vi "GEOM_VAR_RequestedROIsArray.vi"(9 "Action":T2, 10 "ROIs":T1[](array[typedef])) -> (2 "ROIs out":T1[](array[typedef]))   [LabVIEW 2016]
uses:
  GEOM_VAR_action.ctl
  GEOM_Coords.ctl
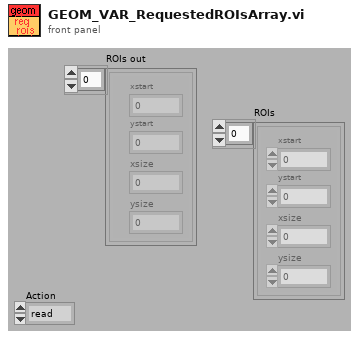
[diagram p1: front panel]
types:
  T1 = typedef "GEOM_Coords.ctl" = cluster{"xstart":u32, "ystart":u32, "xsize":u32, "ysize":u32}
  T2 = typedef "GEOM_VAR_action.ctl" = enum16{"read", "write"}
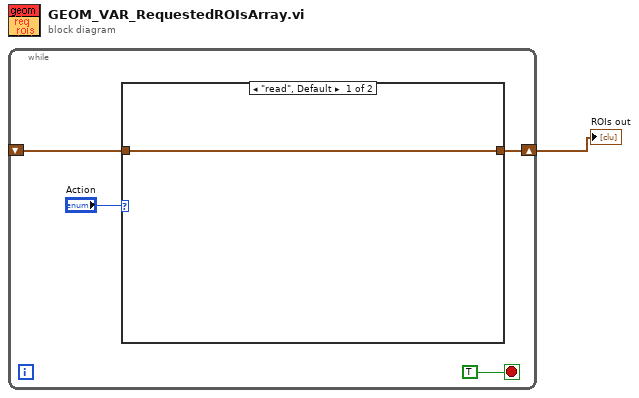
[diagram p0: block diagram]
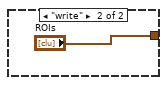
[diagram p2: hidden frame]
diagram:
  n1 = while {
    shift-right: [w2] -> w1
    shift-left: _ -> [w4]
    stop <- TRUE stop-if-true
    n2 = case shown="\"read\", Default" "Action" {
      tunnel: w4 -> [w6 _]
      tunnel: [w6 "ROIs"] -> w2
      frame "read", Default {
      }
      frame "write" {
      }
    }
  }
  "ROIs out" <- w1
